vi "SCLN_PrependSize.vi"(0 "data":string) -> (1 "data with size":string, 2 "error out":errorcluster)   [LabVIEW 2015]
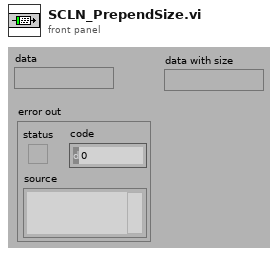
[diagram p1: front panel]
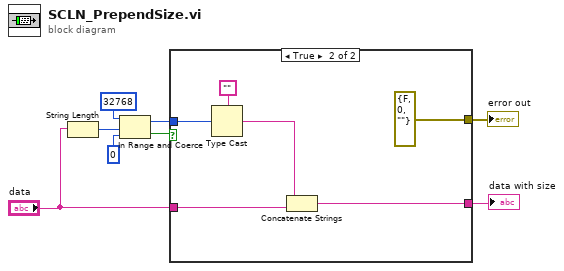
[diagram p0: block diagram]
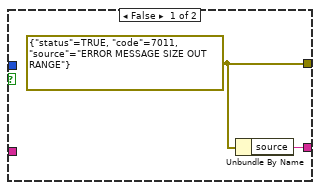
[diagram p2: hidden frame]
diagram:
  n1 = String Length(string="data") -> (length=w5:i32)
  n2 = In Range and Coerce(upper limit=32768, x=w5, lower limit=0) -> (coerced(x)=w3:i32, In Range?=w4:bool)
  n3 = case shown="True" w4 {
    tunnel: "data" -> [_ w15]
    tunnel: w3 -> [_ w14]
    tunnel: [w9 w13] -> w2
    tunnel: [w10 errorcluster {"status"=FALSE, "code"=0, "source"=""} ("error out")] -> w1
    frame False {
      w10 = errorcluster {"status"=TRUE, "code"=7011, "source"="ERROR MESSAGE SIZE OUT RANGE"} ("error out")
      n4 = Unbundle By Name(w10) -> ("source"=w9:string)
    }
    frame True {
      n5 = Type Cast(type="", x=w14) -> (*(type *) &x=w16:string)
      n6 = Concatenate Strings(w16, w15) -> (w13:string)
    }
  }
  "data with size" <- w2
  "error out" <- w1
